vi "closeShutter.vi"(8 "Error In":errorcluster) -> (0 "Error Out":errorcluster)   [LabVIEW 2014]
doc: "Newport Motion Controler\nClose Shutter communication port\n\nAndré Romero - 2022\nandretec@ifsc.usp.br"
uses:
  Global Shutter.vi
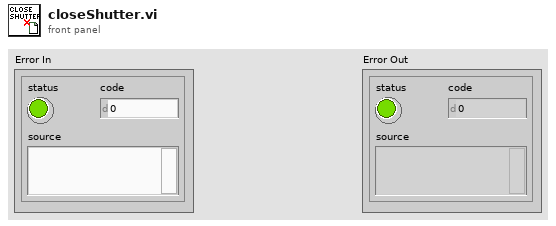
[diagram p1: front panel]
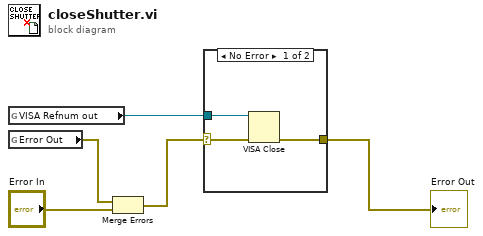
[diagram p0: block diagram]
diagram:
  n1 = global read "Global Shutter.vi" "VISA Refnum out"() -> (w5:refnum<visa-resource-name>)
  n2 = global read "Global Shutter.vi" "Error Out"() -> (w3:errorcluster)
  n3 = Merge Errors(w3, "Error In") -> (w2:errorcluster)
  n4 = case shown="No Error" w2 {
    selector: w2 -> [w7 w9]
    tunnel: w5 -> [w8 _]
    tunnel: [w6 w9] -> w1
    frame No Error {
      n5 = VISA Close(VISA resource name=w8, error in (no error)=w7) -> (error out=w6:errorcluster)
    }
    frame Error {
    }
  }
  "Error Out" <- w1
